vi "ProcessRepository.vi"(0 "reference in":refnum<class "TestView_Base.lvclass">, 1 "Action(ReadRepository)":T1(ring), 5 "error in (no error)":errorcluster) -> (9 "ProcessViRef":refnum<vi>, 11 "ProcessSyncQueue":refnum<queue>, 13 "FromProcessQueue":refnum<queue>, 14 "reference out":refnum<class "TestView_Base.lvclass">, 15 "ToProcessQueue":refnum<queue>, 17 "ProcessAlreadyStarted":bool, 19 "error out":errorcluster)   [LabVIEW 2017]
uses:
  Process.ctl
  TestView_Base.lvclass
  C:/Projects/Audinate/Src/Components/ViPER.lvlibp/ViPER.lvclass
panel:
  # "Use this indicator for sending messages to the Process VI"
  # "These indicators are used by the process VIs"
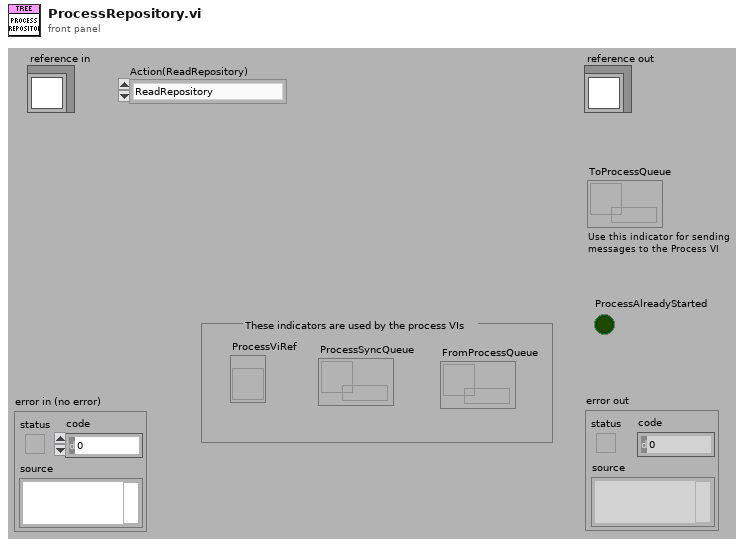
[diagram p1: front panel]
types:
  T1 = enum16{"ReadRepository", "CreateNew", "CreateOrLookUpExisting"}
  T2 = typedef "Process.ctl" = cluster{"ToProcessQueue":refnum<queue>, "FromProcessQueue":refnum<queue>, "ProcessSyncQueue":refnum<queue>, "ProcessViRef":refnum<vi>}
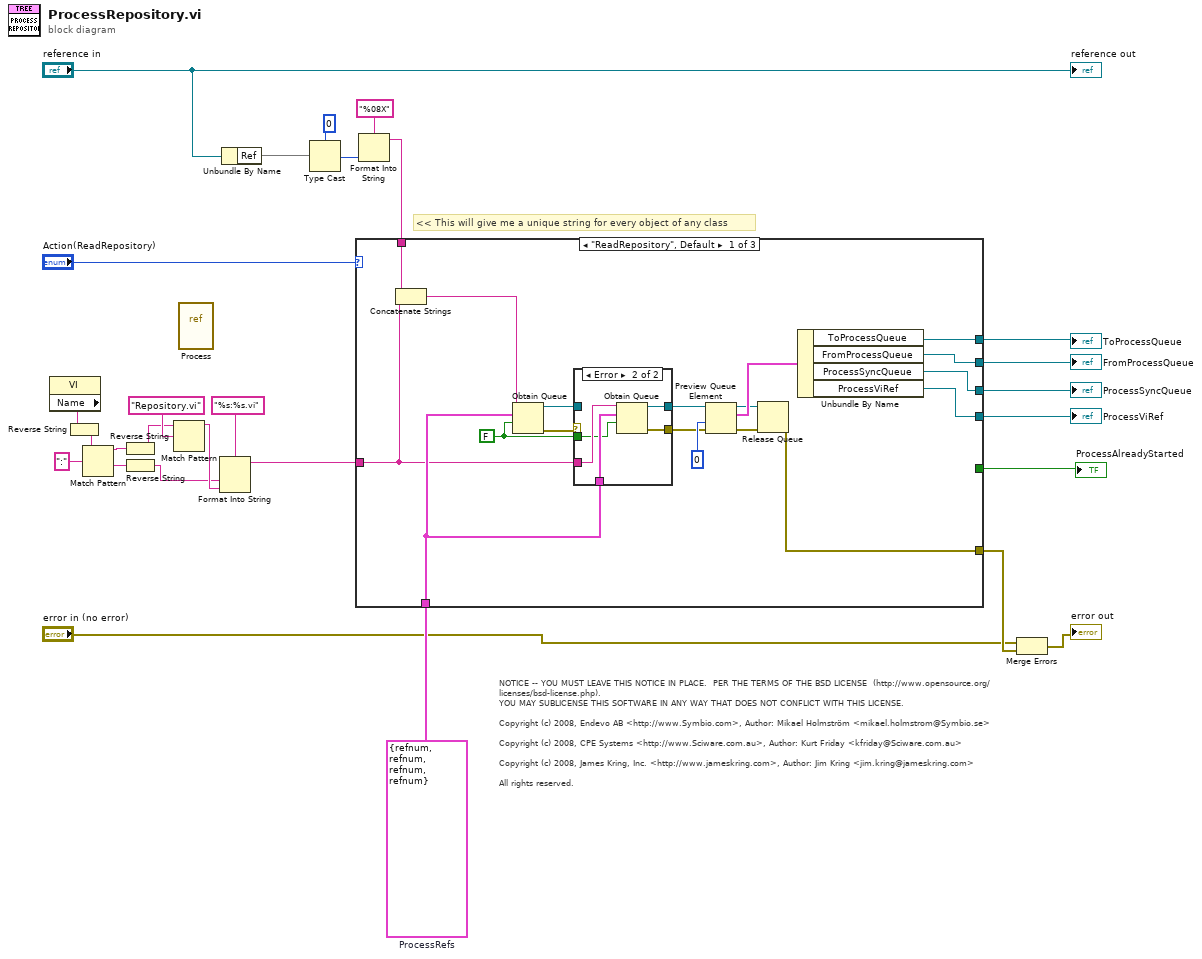
[diagram p0: block diagram]
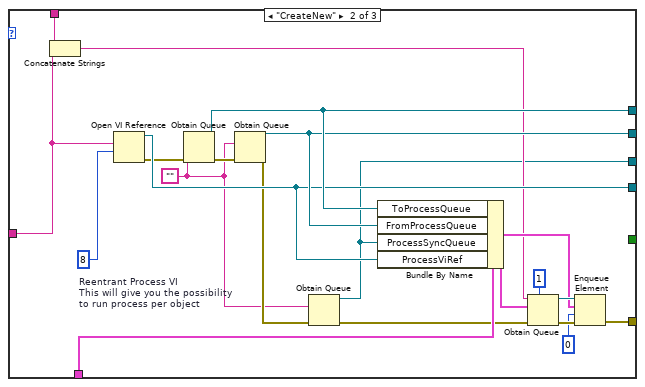
[diagram p3: hidden frame]
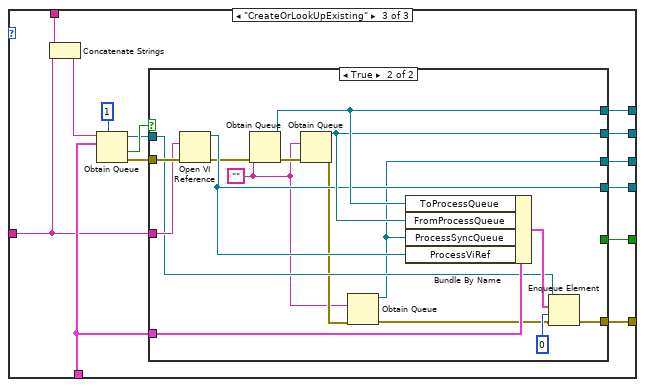
[diagram p4: hidden frame]
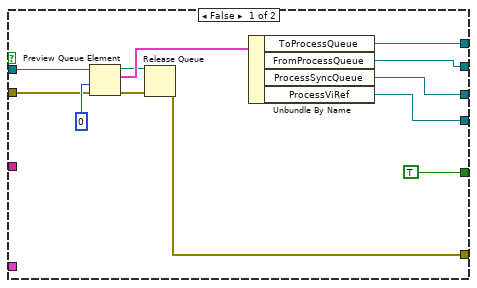
[diagram p5: hidden frame]
diagram:
  w22 = T2 {"ToProcessQueue"=refnum, "FromProcessQueue"=refnum, "ProcessSyncQueue"=refnum, "ProcessViRef"=refnum}  # ProcessRefs
  # "NOTICE -- YOU MUST LEAVE THIS NOTICE IN PLACE.  PER THE TERMS OF THE BSD LICENSE  (http://www.opensource.org/licenses/bsd-license.php).\nYOU MAY SUBLICENSE THIS SOFTWARE IN ANY WAY THAT DOES NOT CONFLICT WITH THIS LICENSE.\n\nCopyright (c) 2008, Endevo AB <http://www.Symbio.com>, Author: Mikael Holmström <mikael.holmstrom@Symbio.se>\n\nCopyright (c) 2008, CPE Systems <http://www.Sciware.com.au>, Author: Kurt Friday <kfriday@Sciware.com.au>\n\nCopyright (c) 2008, James Kring, Inc. <http://www.jameskring.com>, Author: Jim Kring <jim.kring@jameskring.com>\n\nAll rights reserved."
  # "<< This will give me a unique string for every object of any class"
  n1 = property class="VI"() -> ("Name"=w11:string)  [unwired: 2 in, 2 out]
  n2 = Reverse String(1:w11) -> (0:w12:string)
  n3 = Match Pattern(string=w12, regular expression=":") -> (before substring=w16:string, after substring=w13:string)  [unwired: 1 in, 2 out]
  n4 = Reverse String(1:w16) -> (0:w17:string)
  n5 = Reverse String(1:w13) -> (0:w15:string)
  n6 = Match Pattern(string=w17, regular expression="Repository.vi") -> (before substring=w19:string)  [unwired: 1 in, 3 out]
  n7 = vi-ref "Process.vi"() -> ()  [unwired: 1 out]
  n8 = Format Into String(format string="%s:%s.vi", w15, w19) -> (resulting string=w9:string)  [unwired: 2 in, 1 out]
  n9 = Unbundle By Name("reference in") -> ("Ref"=w1)
  n10 = Type Cast(type=u32 0, x=w1) -> (*(type *) &x=w6:u32)
  n11 = Format Into String(format string="%08X", w6) -> (resulting string=w3:string)  [unwired: 2 in, 1 out]
  n12 = case shown="\"ReadRepository\", Default" "Action(ReadRepository)" {
    tunnel: [w40 w54 w84] -> w26
    tunnel: [w42 w72 w86] -> w24
    tunnel: [w41 w71 w85] -> w25
    tunnel: [w43 w70 w83] -> w23
    tunnel: w22 -> [w35 w60 w79]
    tunnel: w3 -> [w33 w59 w75]
    tunnel: [w28 w69 w82] -> w20
    tunnel: w9 -> [w32 w57 w74]
    tunnel: [_ _ w77] -> w8
    frame "ReadRepository", Default {
      w34 = FALSE ("create if not found? (T)")
      n13 = Concatenate Strings(w33, w32) -> (w31:string)
      n14 = Obtain Queue(name (unnamed)=w31, element data type=w35, create if not found? (T)=w34) -> (queue out=w37:refnum<queue>, error out=w39:errorcluster)  [unwired: 2 in, 1 out]
      n15 = case shown="Error" w39 {
        selector: w39 -> [w47 _]
        tunnel: [w47 w49] -> w38
        tunnel: w37 -> [w46 _]
        tunnel: [w46 w50] -> w36
        tunnel: w35 -> [_ w52]
        tunnel: w32 -> [_ w51]
        tunnel: w34 -> [_ w48]
        frame No Error {
        }
        frame Error {
          n16 = Obtain Queue(name (unnamed)=w51, element data type=w52, create if not found? (T)=w48) -> (queue out=w50:refnum<queue>, error out=w49:errorcluster)  [unwired: 2 in, 1 out]
        }
      }
      n17 = Preview Queue Element(queue=w36, timeout in ms (-1)=0, error in (no error)=w38) -> (queue out=w30:refnum<queue>, element=w44:T2, error out=w29:errorcluster)  [unwired: 1 out]
      n18 = Release Queue(queue=w30, error in (no error)=w29) -> (error out=w28:errorcluster)  [unwired: 1 in, 2 out]
      n19 = Unbundle By Name(w44) -> ("ToProcessQueue"=w42:refnum<queue>, "FromProcessQueue"=w41:refnum<queue>, "ProcessSyncQueue"=w40:refnum<queue>, "ProcessViRef"=w43:refnum<vi>)
    }
    frame "CreateNew" {
      w66 = 8  # Reentrant Process VI This will give you the possibility to run process per object
      w53 = ""
      n20 = Concatenate Strings(w59, w57) -> (w58:string)
      n21 = Open VI Reference(vi path=w57, options=w66) -> (vi reference=w70:refnum<vi>, error out=w67:errorcluster)  [unwired: 4 in]
      n22 = Obtain Queue(element data type=w53, error in (no error)=w67) -> (queue out=w72:refnum<queue>, error out=w68:errorcluster)  [unwired: 3 in, 1 out]
      n23 = Obtain Queue(element data type=w53, error in (no error)=w68) -> (queue out=w71:refnum<queue>, error out=w56:errorcluster)  [unwired: 3 in, 1 out]
      n24 = Obtain Queue(element data type=w53, error in (no error)=w56) -> (queue out=w54:refnum<queue>, error out=w55:errorcluster)  [unwired: 3 in, 1 out]
      n25 = Bundle By Name(cluster=w60, "ToProcessQueue"=w72, "FromProcessQueue"=w71, "ProcessSyncQueue"=w54, "ProcessViRef"=w70) -> (w63:T2)
      n26 = Obtain Queue(max queue size (-1, unlimited)=1, name (unnamed)=w58, element data type=w63, error in (no error)=w55) -> (queue out=w65:refnum<queue>, error out=w64:errorcluster)  [unwired: 1 in, 1 out]
      n27 = Enqueue Element(queue=w65, element=w63, timeout in ms (-1)=0, error in (no error)=w64) -> (error out=w69:errorcluster)  [unwired: 2 out]
    }
    frame "CreateOrLookUpExisting" {
      n28 = Concatenate Strings(w75, w74) -> (w73:string)
      n29 = Obtain Queue(max queue size (-1, unlimited)=1, name (unnamed)=w73, element data type=w79) -> (queue out=w80:refnum<queue>, created new?=w81:bool, error out=w78:errorcluster)  [unwired: 2 in]
      n30 = case shown="True" w81 {
        tunnel: [w98 w114] -> w86
        tunnel: [w97 w113] -> w85
        tunnel: [w96 w99] -> w84
        tunnel: [w95 w112] -> w83
        tunnel: [w87 w111] -> w82
        tunnel: w79 -> [_ w110]
        tunnel: w78 -> [w92 w105]
        tunnel: w74 -> [_ w104]
        tunnel: w80 -> [w93 w103]
        tunnel: [TRUE _] -> w77
        frame False {
          n31 = Preview Queue Element(queue=w93, timeout in ms (-1)=0, error in (no error)=w92) -> (queue out=w89:refnum<queue>, element=w91:T2, error out=w88:errorcluster)  [unwired: 1 out]
          n32 = Release Queue(queue=w89, error in (no error)=w88) -> (error out=w87:errorcluster)  [unwired: 1 in, 2 out]
          n33 = Unbundle By Name(w91) -> ("ToProcessQueue"=w98:refnum<queue>, "FromProcessQueue"=w97:refnum<queue>, "ProcessSyncQueue"=w96:refnum<queue>, "ProcessViRef"=w95:refnum<vi>)
        }
        frame True {
          w100 = ""
          n34 = Open VI Reference(vi path=w104, error in (no error)=w105) -> (vi reference=w112:refnum<vi>, error out=w108:errorcluster)  [unwired: 4 in]
          n35 = Obtain Queue(element data type=w100, error in (no error)=w108) -> (queue out=w114:refnum<queue>, error out=w109:errorcluster)  [unwired: 3 in, 1 out]
          n36 = Obtain Queue(element data type=w100, error in (no error)=w109) -> (queue out=w113:refnum<queue>, error out=w102:errorcluster)  [unwired: 3 in, 1 out]
          n37 = Obtain Queue(element data type=w100, error in (no error)=w102) -> (queue out=w99:refnum<queue>, error out=w101:errorcluster)  [unwired: 3 in, 1 out]
          n38 = Bundle By Name(cluster=w110, "ToProcessQueue"=w114, "FromProcessQueue"=w113, "ProcessSyncQueue"=w99, "ProcessViRef"=w112) -> (w107:T2)
          n39 = Enqueue Element(queue=w103, element=w107, timeout in ms (-1)=0, error in (no error)=w101) -> (error out=w111:errorcluster)  [unwired: 2 out]
        }
      }
    }
  }
  "ProcessSyncQueue" <- w26
  "ToProcessQueue" <- w24
  "FromProcessQueue" <- w25
  "ProcessViRef" <- w23
  "ProcessAlreadyStarted" <- w8
  n40 = Merge Errors("error in (no error)", w20) -> (→"error out":errorcluster)
  "reference out" <- "reference in"
